vi "Wrap In Generic.vi"(8 "error in (no error)":errorcluster, 11 "Data to Wrap":variant) -> (0 "error out":errorcluster, 3 "Generic Data":refnum<class "Generic Data.lvclass">)   [LabVIEW 2020, in "Data.lvlib"]
doc: "Wrap the data from 'Data to Wrap' in a Generic class instance."
uses:
  Data.lvlib
  Generic Data/Generic Data.lvclass
  Generic Data/I32/I32.lvclass/I32.ctl
  Generic Data/Waveform/Waveform.lvclass/Waveform.ctl
  Generic Data/U32/U32.lvclass/U32.ctl
  Generic Data/Generic Array Data/I32 Array/I32 Array.lvclass/I32 Array.ctl
  Generic Data/Generic Array Data/U32 Array/U32 Array.lvclass/U32 Array.ctl
  Generic Data/Generic Array Data/Double Array/Double Array.lvclass/Double Array.ctl
  Generic Data/Generic Array Data/Boolean Array/Boolean Array.lvclass/Boolean Array.ctl
  Generic Data/Generic Array Data/Waveform Array/Waveform Array.lvclass/Waveform Array.ctl
  Generic Data/Generic Array Data/String Array/String Array.lvclass/String Array.ctl
  Generic Data/Generic Array Data/Path Array/Path Array.lvclass/Path Array.ctl
  Generic Data/Generic Array Data/Time Stamp Array/Time Stamp Array.lvclass/Time Stamp Array.ctl
  Generic Data/Data Class/Data Class.lvclass
  C:/Users/Henri/OneDrive/LabVIEW/Framework/Data/Generic Data/Generic Data.lvclass
  Generic Data/Double/Double.lvclass/Double.ctl
  Generic Data/Boolean/Boolean.lvclass/Boolean.ctl
  Data.lvclass
  Generic Data/String/String.lvclass/String.ctl
  Generic Data/Path/Path.lvclass/Path.ctl
  Generic Data/Time Stamp/Time Stamp.lvclass/Time Stamp.ctl
  Generic Data/Variant/Variant.lvclass/Variant.ctl
  Generic Data/I32/I32.lvclass
  Generic Data/Waveform/Waveform.lvclass
  Generic Data/U32/U32.lvclass
  Generic Data/Double/Double.lvclass
  Generic Data/Boolean/Boolean.lvclass
  Generic Data/Cluster/Cluster.lvclass
  Generic Data/String/String.lvclass
  Generic Data/Path/Path.lvclass
  Generic Data/Time Stamp/Time Stamp.lvclass
  Generic Data/Enum/Enum.lvclass
  Generic Data/Generic Array Data/I32 Array/I32 Array.lvclass
  Generic Data/Generic Array Data/U32 Array/U32 Array.lvclass
  Generic Data/Generic Array Data/Double Array/Double Array.lvclass
  Generic Data/Generic Array Data/Boolean Array/Boolean Array.lvclass
  Generic Data/Generic Array Data/Waveform Array/Waveform Array.lvclass
  Generic Data/Generic Array Data/String Array/String Array.lvclass
  Generic Data/Generic Array Data/Path Array/Path Array.lvclass
  Generic Data/Generic Array Data/Time Stamp Array/Time Stamp Array.lvclass
  Generic Data/Generic Array Data/Data Class Array/Data Class Array.lvclass
  Generic Data/Generic Array Data/Cluster Array/Cluster Array.lvclass
  Generic Data/Generic Array Data/Enum Array/Enum Array.lvclass
  Generic Data/Variant/Variant.lvclass
  <vilib>/Utility/Data Type/NI_Data Type.lvlib
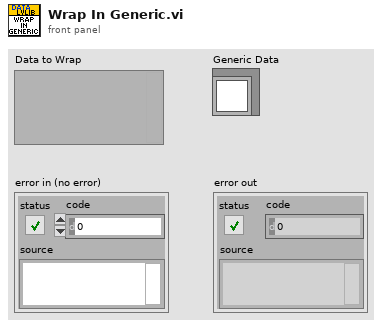
[diagram p1: front panel]
types:
  T1 = typedef "NI_Data Type.lvlib/Data Type.ctl" = enum8{"Invalid Type", "Void", "I8", "I16", "I32", "I64", "U8", "U16", "U32", "U64", "Single Float", "Double Float", "Extended Float", "Single Complex", "Double Complex", "Extended Complex", "Enum U8", "Enum U16", "Enum U32", "Enum U64", "Single Float With Unit", "Double Float With Unit", "Extended Float With Unit", "Single Complex with Unit", "Double Complex with Unit", "Extended Complex with Unit", "Boolean", "String", "Path", "Picture", "Tag", "Array", "Cluster", "Variant", "LV Variant", "Waveform", "Timestamp", "Digital Waveform", "Digital Data", "ExpressData", "Refnum", "External Data", "VI", "Poly VI", "LabVIEW Class Instance", "Fixed Point", "Set Collection", "Map Collection"}
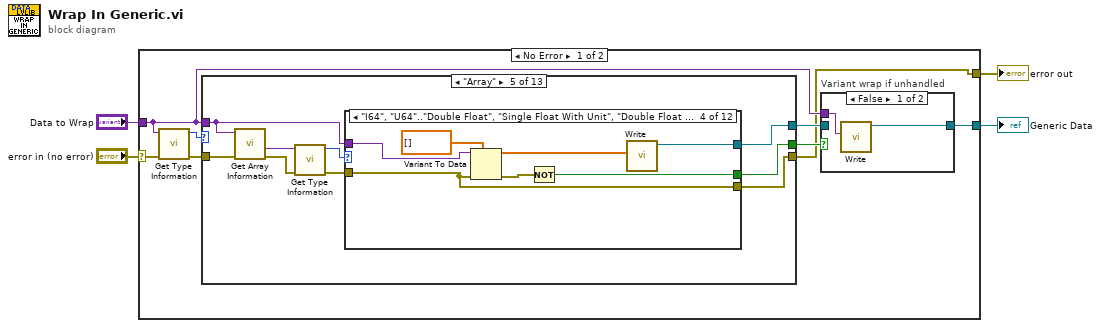
[diagram p0: block diagram]
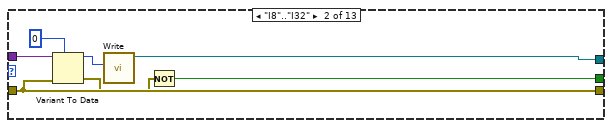
[diagram p4: hidden frame]
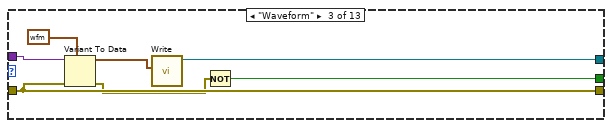
[diagram p5: hidden frame]
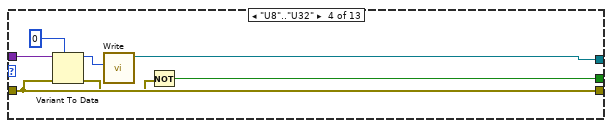
[diagram p6: hidden frame]
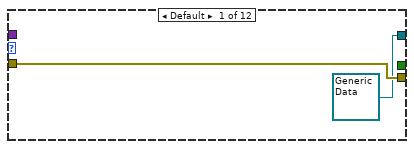
[diagram p7: hidden frame]
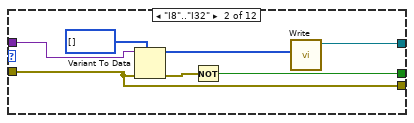
[diagram p8: hidden frame]
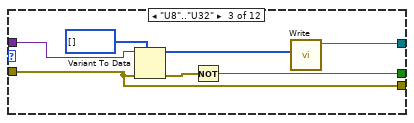
[diagram p9: hidden frame]
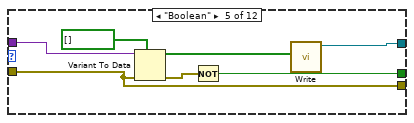
[diagram p10: hidden frame]
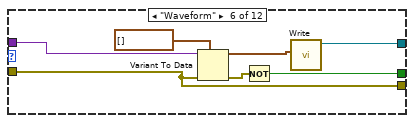
[diagram p11: hidden frame]
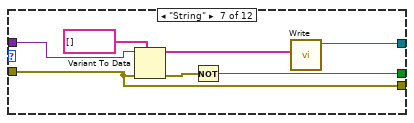
[diagram p12: hidden frame]
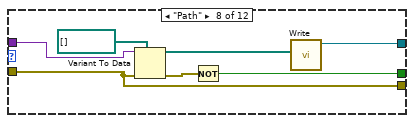
[diagram p13: hidden frame]
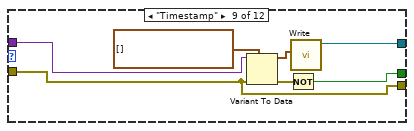
[diagram p14: hidden frame]
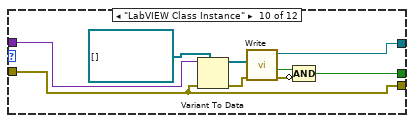
[diagram p15: hidden frame]
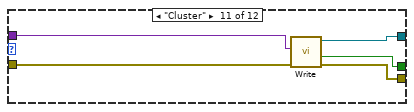
[diagram p16: hidden frame]
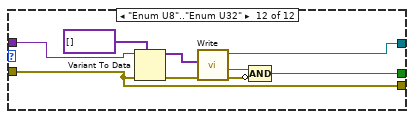
[diagram p17: hidden frame]
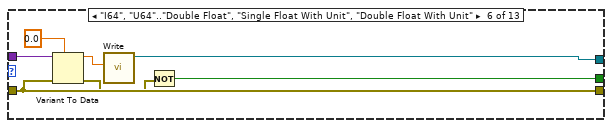
[diagram p18: hidden frame]
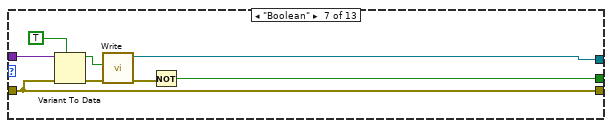
[diagram p19: hidden frame]
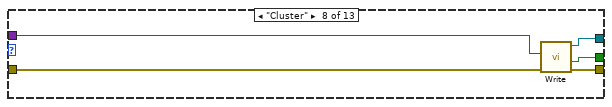
[diagram p20: hidden frame]
diagram:
  n1 = case shown="No Error" "error in (no error)" {
    selector: "error in (no error)" -> [w12 w185]
    tunnel: "Data to Wrap" -> [w6 _]
    tunnel: [w8 _] -> w2
    tunnel: [w5 w185] -> w1
    frame No Error {
      n2 = call <vilib>:"Get Type Information.vi"("error in (no error)"=w12, "variant"=w6) -> ("error out"=w10:errorcluster, "type"=w11:T1)  [unwired: 5 in, 3 out]
      n3 = case shown="\"Array\"" w11 {
        tunnel: w6 -> [_ w23 w30 w37 w43 w134 w141 w146 w149 w165 w172 w179 w184]
        tunnel: w10 -> [w16 w18 w26 w32 w45 w129 w138 w143 w150 w162 w169 w176 w181]
        tunnel: [_ w20 w28 w34 w40 w131 w140 w145 w152 w164 w171 w178 w182] -> w7
        tunnel: [_ w19 w27 w33 w38 w130 w139 w144 w153 w163 w170 w177 w183] -> w9
        tunnel: [w16 w18 w26 w32 w39 w129 w138 w142 w150 w162 w169 w176 w180] -> w5
        frame Default {
        }
        frame "I8".."I32" {
          n4 = Variant To Data(error in=w18, type=0 ("I32"), Variant=w23) -> (data=w21:i32, error out=w17:errorcluster)
          n5 = call "Write.vi"("I32"=w21) -> ("I32 out"=w20:refnum<class "I32.lvclass">)  [unwired: 10 in]
          n6 = Not(x=w17) -> (.not. x?=w19:bool)
        }
        frame "Waveform" {
          n7 = Variant To Data(error in=w26, type=waveform(dbl) {"t0"=timestamp(0 s since 1904-01-01), "dt"=1.0, "Y"=[]}, Variant=w30) -> (data=w25:waveform(dbl), error out=w24:errorcluster)
          n8 = call "Write.vi"("Waveform"=w25) -> ("Waveform out"=w28:refnum<class "Waveform.lvclass">)  [unwired: 10 in]
          n9 = Not(x=w24) -> (.not. x?=w27:bool)
        }
        frame "U8".."U32" {
          n10 = Variant To Data(error in=w32, type=u32 0 ("I32"), Variant=w37) -> (data=w35:u32, error out=w31:errorcluster)
          n11 = call "Write.vi"("U32"=w35) -> ("U32 out"=w34:refnum<class "U32.lvclass">)  [unwired: 10 in]
          n12 = Not(x=w31) -> (.not. x?=w33:bool)
        }
        frame "Array" {
          n13 = call <vilib>:"Get Array Information.vi"("error in (no error)"=w45, "variant"=w43) -> ("error out"=w44:errorcluster, "array element data type"=w46:variant)  [unwired: 6 in, 2 out]
          n14 = call <vilib>:"Get Type Information.vi"("error in (no error)"=w44, "variant"=w46) -> ("error out"=w42:errorcluster, "type"=w41:T1)  [unwired: 5 in, 3 out]
          n15 = case shown="\"I64\", \"U64\"..\"Double Float\", \"Single Float With Unit\", \"Double Float With Unit\"" w41 {
            tunnel: w43 -> [_ w55 w62 w69 w76 w83 w90 w97 w104 w113 w118 w127]
            tunnel: w42 -> [w48 w50 w57 w64 w73 w81 w87 w94 w101 w112 w115 w121]
            tunnel: [refnum<class "Generic Data.lvclass"> refnum ("U32 out") w52 w59 w66 w75 w78 w89 w96 w103 w105 w117 w122] -> w40
            tunnel: [_ w51 w58 w65 w74 w82 w88 w95 w102 w107 w116 w123] -> w38
            tunnel: [w48 w50 w57 w64 w73 w81 w87 w94 w101 w112 w114 w121] -> w39
            frame Default {
            }
            frame "I8".."I32" {
              n16 = Variant To Data(error in=w50, type=i32[] [] ("I32"), Variant=w55) -> (data=w53:i32[], error out=w49:errorcluster)
              n17 = Not(x=w49) -> (.not. x?=w51:bool)
              n18 = call "Write.vi"("I32 Array"=w53) -> ("I32 Array out"=w52:refnum<class "I32 Array.lvclass">)  [unwired: 10 in]
            }
            frame "U8".."U32" {
              n19 = Variant To Data(error in=w57, type=u32[] [] ("I32"), Variant=w62) -> (data=w60:u32[], error out=w56:errorcluster)
              n20 = Not(x=w56) -> (.not. x?=w58:bool)
              n21 = call "Write.vi"("U32 Array"=w60) -> ("U32 Array out"=w59:refnum<class "U32 Array.lvclass">)  [unwired: 10 in]
            }
            frame "I64", "U64".."Double Float", "Single Float With Unit", "Double Float With Unit" {
              n22 = Variant To Data(error in=w64, type=dbl[] [] ("I32"), Variant=w69) -> (data=w67:dbl[], error out=w63:errorcluster)
              n23 = Not(x=w63) -> (.not. x?=w65:bool)
              n24 = call "Write.vi"("Double Array"=w67) -> ("Double Array out"=w66:refnum<class "Double Array.lvclass">)  [unwired: 10 in]
            }
            frame "Boolean" {
              n25 = Variant To Data(error in=w73, type=bool[] [], Variant=w76) -> (data=w71:bool[], error out=w70:errorcluster)
              n26 = Not(x=w70) -> (.not. x?=w74:bool)
              n27 = call "Write.vi"("Boolean Array"=w71) -> ("Boolean Array out"=w75:refnum<class "Boolean Array.lvclass">)  [unwired: 10 in]
            }
            frame "Waveform" {
              n28 = Variant To Data(error in=w81, type=waveform(dbl)[] [], Variant=w83) -> (data=w79:waveform(dbl)[], error out=w77:errorcluster)
              n29 = Not(x=w77) -> (.not. x?=w82:bool)
              n30 = call "Write.vi"("Waveform Array"=w79) -> ("Waveform Array out"=w78:refnum<class "Waveform Array.lvclass">)  [unwired: 10 in]
            }
            frame "String" {
              n31 = Variant To Data(error in=w87, type=string[] [], Variant=w90) -> (data=w85:string[], error out=w84:errorcluster)
              n32 = Not(x=w84) -> (.not. x?=w88:bool)
              n33 = call "Write.vi"("String Array"=w85) -> ("String Array out"=w89:refnum<class "String Array.lvclass">)  [unwired: 10 in]
            }
            frame "Path" {
              n34 = Variant To Data(error in=w94, type=path[] [], Variant=w97) -> (data=w92:path[], error out=w91:errorcluster)
              n35 = Not(x=w91) -> (.not. x?=w95:bool)
              n36 = call "Write.vi"("Path Array"=w92) -> ("Path Array out"=w96:refnum<class "Path Array.lvclass">)  [unwired: 10 in]
            }
            frame "Timestamp" {
              n37 = Variant To Data(error in=w101, type=timestamp[] [], Variant=w104) -> (data=w99:timestamp[], error out=w98:errorcluster)
              n38 = Not(x=w98) -> (.not. x?=w102:bool)
              n39 = call "Write.vi"("String Array"=w99) -> ("String Array out"=w103:refnum<class "Time Stamp Array.lvclass">)  [unwired: 10 in]
            }
            frame "LabVIEW Class Instance" {
              n40 = Variant To Data(error in=w112, type=refnum<class "Data Class.lvclass">[] [], Variant=w113) -> (data=w106:refnum<class "Data Class.lvclass">[], error out=w110:errorcluster)
              n41 = call "Write.vi"("error in (no error)"=w110, "Data Class Array"=w106) -> ("error out"=w108:errorcluster, "Success?"=w109:bool, "Data Class Array out"=w105:refnum<class "Data Class Array.lvclass">)  [unwired: 7 in]
              n42 = Compound Arithmetic op=AND(w109, invert w108) -> (w107:bool)
            }
            frame "Cluster" {
              n43 = call "Write.vi"("error in (no error)"=w115, "Cluster Array"=w118) -> ("error out"=w114:errorcluster, "Success?"=w116:bool, "Cluster Array out"=w117:refnum<class "Cluster Array.lvclass">)  [unwired: 7 in]
            }
            frame "Enum U8".."Enum U32" {
              n44 = Variant To Data(error in=w121, type=variant[] [], Variant=w127) -> (data=w124:variant[], error out=w120:errorcluster)
              n45 = call "Write.vi"("error in (no error)"=w120, "Enum Variant"=w124) -> ("error out"=w119:errorcluster, "Success?"=w126:bool, "Enum Array out"=w122:refnum<class "Enum Array.lvclass">)  [unwired: 7 in]
              n46 = Compound Arithmetic op=AND(w126, invert w119) -> (w123:bool)
            }
          }
        }
        frame "I64", "U64".."Double Float", "Single Float With Unit", "Double Float With Unit" {
          n47 = Variant To Data(error in=w129, type=0.0 ("I32"), Variant=w134) -> (data=w132:dbl, error out=w128:errorcluster)
          n48 = call "Write.vi"("Double"=w132) -> ("Double out"=w131:refnum<class "Double.lvclass">)  [unwired: 10 in]
          n49 = Not(x=w128) -> (.not. x?=w130:bool)
        }
        frame "Boolean" {
          n50 = Variant To Data(error in=w138, type=TRUE, Variant=w141) -> (data=w136:bool, error out=w135:errorcluster)
          n51 = call "Write.vi"("Boolean"=w136) -> ("Boolean out"=w140:refnum<class "Boolean.lvclass">)  [unwired: 10 in]
          n52 = Not(x=w135) -> (.not. x?=w139:bool)
        }
        frame "Cluster" {
          n53 = call "Write.vi"("error in (no error)"=w143, "Cluster"=w146) -> ("error out"=w142:errorcluster, "Success?"=w144:bool, "Cluster out"=w145:refnum<class "Cluster.lvclass">)  [unwired: 7 in]
        }
        frame "LabVIEW Class Instance" {
          n54 = Variant To Data(error in=w150, type=refnum<class "Data.lvclass"> refnum ("Data"), Variant=w149) -> (data=w147:refnum<class "Data.lvclass">, error out=w151:errorcluster)
          n55 = case shown="No Error" w151 {
            selector: w151 -> [w155 _]
            tunnel: [w157 _] -> w153
            tunnel: [w156 _] -> w152
            tunnel: w147 -> [w154 _]
            frame No Error {
              n56 = call "Write.vi"("error in (no error)"=w155, "Data"=w154) -> ("error out"=w158:errorcluster, "Data Class out"=w156:refnum<class "Data Class.lvclass">)  [unwired: 8 in]
              n57 = Not(x=w158) -> (.not. x?=w157:bool)
            }
            frame Error {
            }
          }
        }
        frame "String" {
          n58 = Variant To Data(error in=w162, type="", Variant=w165) -> (data=w160:string, error out=w159:errorcluster)
          n59 = call "Write.vi"("String"=w160) -> ("String out"=w164:refnum<class "String.lvclass">)  [unwired: 10 in]
          n60 = Not(x=w159) -> (.not. x?=w163:bool)
        }
        frame "Path" {
          n61 = Variant To Data(error in=w169, type=path "", Variant=w172) -> (data=w167:path, error out=w166:errorcluster)
          n62 = call "Write.vi"("Path"=w167) -> ("Path out"=w171:refnum<class "Path.lvclass">)  [unwired: 10 in]
          n63 = Not(x=w166) -> (.not. x?=w170:bool)
        }
        frame "Timestamp" {
          n64 = Variant To Data(error in=w176, type=timestamp(0 s since 1904-01-01), Variant=w179) -> (data=w174:timestamp, error out=w173:errorcluster)
          n65 = call "Write.vi"("Time Stamp"=w174) -> ("Time Stamp out"=w178:refnum<class "Time Stamp.lvclass">)  [unwired: 10 in]
          n66 = Not(x=w173) -> (.not. x?=w177:bool)
        }
        frame "Enum U8".."Enum U32" {
          n67 = call "Write.vi"("error in (no error)"=w181, "Enum Variant"=w184) -> ("error out"=w180:errorcluster, "Success?"=w183:bool, "Enum out"=w182:refnum<class "Enum.lvclass">)  [unwired: 7 in]
        }
      }
      n68 = case "Variant wrap if unhandled" shown="False" w9 {
        tunnel: [w13 w15] -> w8
        tunnel: w7 -> [_ w15]
        tunnel: w6 -> [w14 _]
        frame False {
          n69 = call "Write.vi"("Variant"=w14) -> ("Variant out"=w13:refnum<class "Variant.lvclass">)  [unwired: 10 in]
        }
        frame True {
        }
      }
    }
    frame Error {
    }
  }
  "Generic Data" <- w2
  "error out" <- w1
